vi "_FPGA_MovingAverage8elements.vi"(10 "Value in":fxp<+/-,24,5>) -> (2 "Moving average out":fxp<+/-,24,5>)   [LabVIEW 2018]
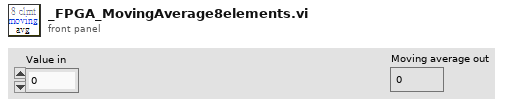
[diagram p1: front panel]
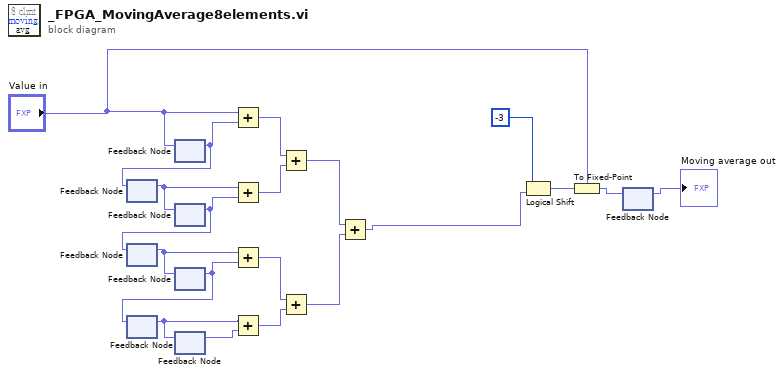
[diagram p0: block diagram]
diagram:
  n1 = feedback #1() -> (w14:fxp<+/-,24,5>)  [unwired: 1 in]
  n2 = feedback #2() -> (w11:fxp<+/-,24,5>)  [unwired: 1 in]
  n3 = feedback #3() -> (w9:fxp<+/-,24,5>)  [unwired: 1 in]
  n4 = feedback #4() -> (w15:fxp<+/-,24,5>)  [unwired: 1 in]
  n5 = feedback-in #1(w15) -> ()
  n6 = feedback-in #4("Value in") -> ()
  n7 = feedback #5() -> (w13:fxp<+/-,24,5>)  [unwired: 1 in]
  n8 = feedback-in #2(w13) -> ()
  n9 = feedback-in #5(w14) -> ()
  n10 = feedback #6() -> (w10:fxp<+/-,24,5>)  [unwired: 1 in]
  n11 = feedback-in #3(w10) -> ()
  n12 = feedback-in #6(w11) -> ()
  n13 = feedback #7() -> (w8:fxp<+/-,24,5>)  [unwired: 1 in]
  n14 = feedback-in #7(w9) -> ()
  n15 = Add(x="Value in", y=w15) -> (x+y=w7:fxp<+/-,25,6>)
  n16 = Add(x=w14, y=w13) -> (x+y=w6:fxp<+/-,25,6>)
  n17 = Add(x=w11, y=w10) -> (x+y=w5:fxp<+/-,25,6>)
  n18 = Add(x=w9, y=w8) -> (x+y=w4:fxp<+/-,25,6>)
  n19 = Add(x=w7, y=w6) -> (x+y=w3:fxp<+/-,26,7>)
  n20 = Add(x=w5, y=w4) -> (x+y=w2:fxp<+/-,26,7>)
  n21 = Add(x=w3, y=w2) -> (x+y=w1:fxp<+/-,27,8>)
  n22 = Logical Shift(y=i16 -3, x=w1) -> (x << y=w18:fxp<+/-,27,8>)
  n23 = To Fixed-Point(fixed-point type="Value in", number=w18) -> (fixed-point=w17:fxp<+/-,24,5>)
  n24 = feedback-in #8(w17) -> ()
  n25 = feedback #8() -> (→"Moving average out":fxp<+/-,24,5>)  [unwired: 1 in]
